vi "FieldController.vi"() -> (3 "Field Controller":u64[](array[numeric]), 5 "error out":errorcluster)   [LabVIEW 2020, in "SnapMB.lvlib"]
uses:
  SnapMB.lvlib
  windows/snapmb.dll
panel:
  in  "error in (no error)":errorcluster
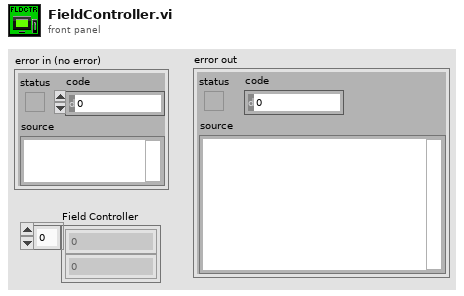
[diagram p1: front panel]
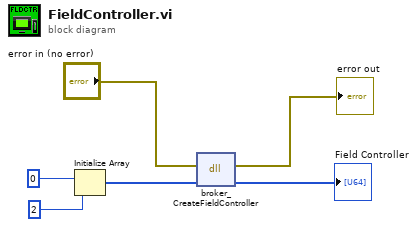
[diagram p0: block diagram]
diagram:
  n1 = Initialize Array(u64 0 ("element"), 2 ("dimension size")) -> (w4:u64[])
  n2 = dll-call lib="D:/SnapMB/LabView/lib/windows/snapmb.dll" fn="broker_CreateFieldController"(error in="error in (no error)", "Broker"=w4) -> (error out=→"error out":errorcluster, "Broker"=→"Field Controller":u64[])  [unwired: 3 in, 1 out]
